vi "Global Variables.vi"() -> ()   [LabVIEW 2014]
panel:
  in  "J-Stk 0 Buttons":string="Joystick 0/Buttons"
  in  "J-Stk 0 Axes":string="Joystick 0/Axes"
  in  "Drive Motors":string="RobotDrive Motors"
  in  "Piston":string="Piston"
  in  "Indexer":string="Indexer"
  in  "Shooter":string="Shooter"
  in  "Joystick 0":string="Joystick 0"
  in  "Motors":string="Left and Right Motors"
  # "Motors"
  # "Joysticks"
  # "Solenoids"
  # "Relays"
  # "Dashboard"
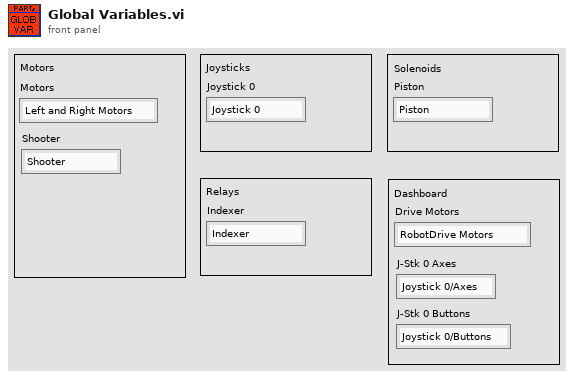
[diagram p1: front panel]
diagram:
